vi "mupExpr Test Exec.vi"() -> ()   [LabVIEW 2015]
uses:
  mupExpr/mupExpr.lvclass/mupExpr.ctl
  mupExpr/Eval.vi
  mupLib/mupSetVarValue.vi
  mupLib/mupEval.vi
  mupLib/mupCheckError.vi
  mupLib/mupLibPath.vi
  <vilib>/Utility/error.llb/Error Cluster From Error Code.vi
  mupExpr/mupExpr.lvclass
panel:
  out "error out":errorcluster
  in  "Iterations":i32=1000
  in  "Plot":bool
  in  "Expression":string="1*x+0"
  out "XY Graph":cluster{dbl[], dbl[]}(graph)
  # "Single Variable \"x\""
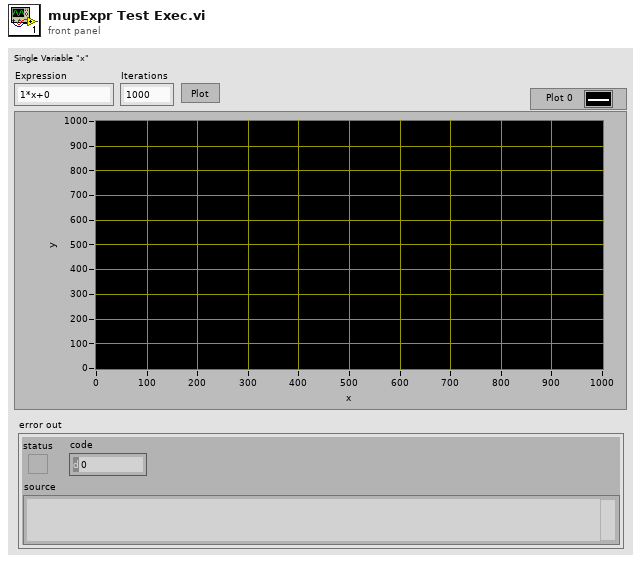
[diagram p1: front panel]
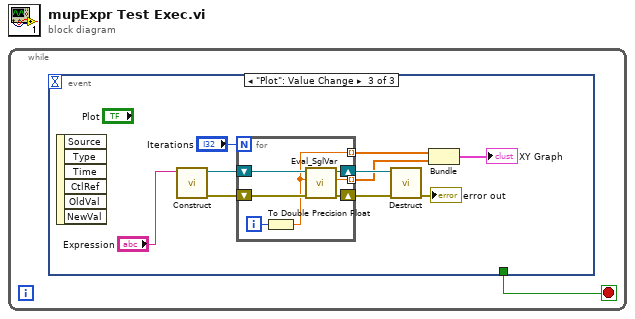
[diagram p0: block diagram]
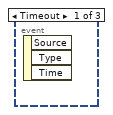
[diagram p2: hidden frame]
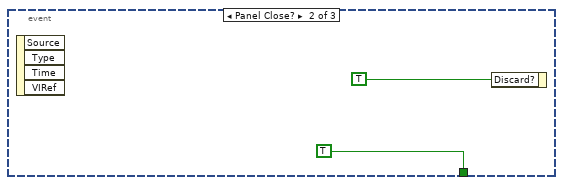
[diagram p3: hidden frame]
diagram:
  n1 = while {
    stop <- w1 stop-if-true
    n2 = event shown="[2] \"Plot\": Value Change" {
      selector: _ -> [_ _ _]
      dyn-events: _ -> [_ _ _]
      timeout: _ -> [_ _ _]
      tunnel: [_ TRUE _] -> w1
      event Timeout {
        n3 = event-data() -> ()  [unwired: 1 in, 3 out]
      }
      event Panel Close? {
        n4 = event-data() -> ()  [unwired: 1 in, 4 out]
        n5 = event-data("Discard?"=TRUE) -> ()  [unwired: 1 in, 1 out]
      }
      event "Plot": Value Change {
        n6 = event-data() -> ()  [unwired: 1 in, 6 out]
        n7 = call "Construct.vi"("Expression"="Expression") -> ("error out"=w12:errorcluster, "muExpr out"=w10:refnum<class "mupExpr.lvclass">)  [unwired: 8 in, 1 out]
        n8 = for {
          N: "Iterations" -> [_]
          shift-right: [w19] -> w11
          shift-left: w10 -> [w20]
          shift-right: [w17] -> w13
          shift-left: w12 -> [w18]
          tunnel: [w15] -> w8 mode=indexing
          tunnel: [w14] -> w9 mode=indexing
          i -> [w16]
          n9 = To Double Precision Float(number=w16) -> (double precision float=w14:dbl)
          n10 = call "Eval_SglVar.vi"("error in (no error)"=w18, "varValue"=w14, "muExpr in"=w20) -> ("error out"=w17:errorcluster, "Result"=w15:dbl, "muExpr out"=w19:refnum<class "mupExpr.lvclass">)  [unwired: 6 in]
        }
        n11 = call "Destruct.vi"("error in (no error)"=w13, "muExpr in"=w11) -> ("error out"=→"error out":errorcluster)  [unwired: 9 in]
        n12 = Bundle(w9, w8) -> (→"XY Graph":cluster{dbl[], dbl[]})  [unwired: 1 in]
      }
    }
  }
